vi "Operator.vi"(8 "error in (no error)":errorcluster, 11 "Logical Or in":refnum<class "Logical Or.lvclass">) -> (0 "error out":errorcluster, 2 "Operator":string, 3 "Logical Or out":refnum<class "Logical Or.lvclass">)   [LabVIEW 2017, in "Transparent Assertions.lvlib" / "Constraints.lvlib" / "Logical Or.lvclass"]
uses:
  Logical Or.lvclass
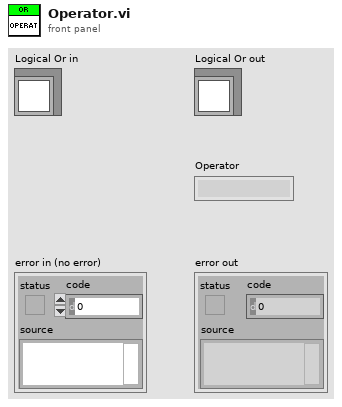
[diagram p1: front panel]
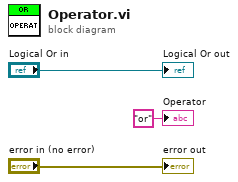
[diagram p0: block diagram]
diagram:
  "error out" <- "error in (no error)"
  "Logical Or out" <- "Logical Or in"
  "Operator" <- "or" ("Operator")
